vi "GetCollisions.vi"(8 "error in":errorcluster, 11 "sprite in":refnum<class "Sprite.lvclass">) -> (0 "error out":errorcluster, 2 "collisions out":string[](array[string]), 3 "sprite out":refnum<class "Sprite.lvclass">)   [LabVIEW 2010, in "RenderBase.lvlib" / "Sprite.lvclass"]
doc: "Returns the names of the objects that currently cause collisions. This is a default implementation that supports 2D collisions only. We also assume that the collisions don't change as long as the sprite's position doesn't change. Override this method if you need something more elaborated."
uses:
  Sprite.lvclass
  Sprite.lvclass/Sprite.ctl
  SceneObject_class/properties/SceneRoot/GetSceneRoot.vi
  SceneObject_class/properties/Position/GetPosition.vi
  SceneRoot_class/SceneRoot.lvclass
  SceneObject_class/SceneObject.lvclass
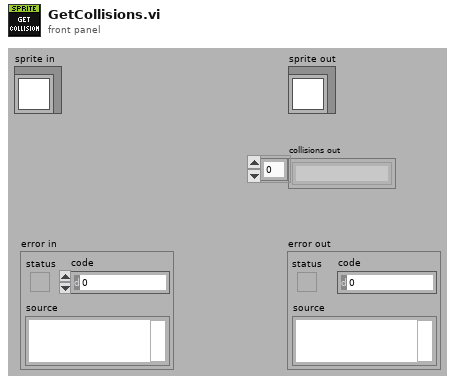
[diagram p1: front panel]
types:
  T1 = typedef "LV3DPointTypeDef.ctl" = cluster{"X":sgl, "Y":sgl, "Z":sgl}
  T2 = typedef "LVPoint32TypeDef.ctl" = cluster{"Horizontal":i32, "Vertical":i32}
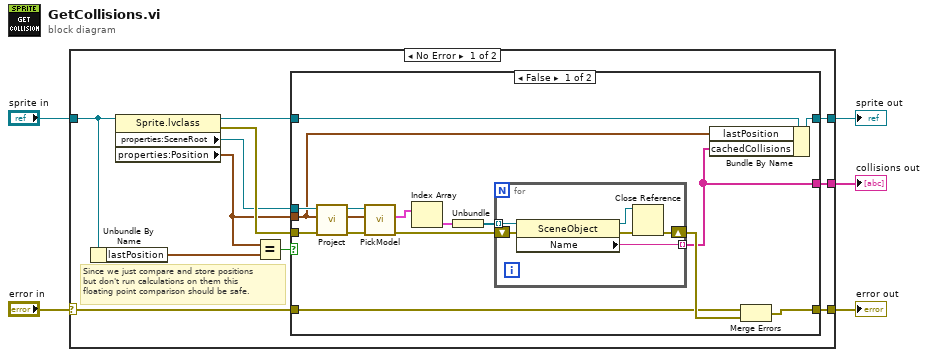
[diagram p0: block diagram]
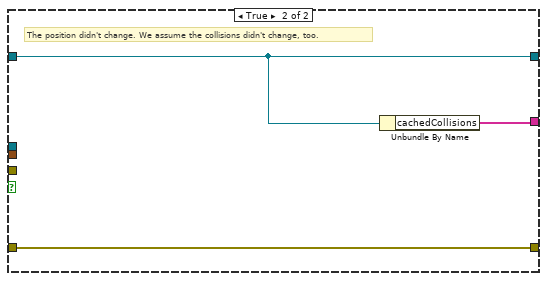
[diagram p2: hidden frame]
diagram:
  n1 = case shown="No Error" "error in" {
    selector: "error in" -> [w14 w43]
    tunnel: "sprite in" -> [w9 w42]
    tunnel: [w15 w43] -> w2
    tunnel: [w10 w42] -> w3
    tunnel: [w16 _] -> w4
    frame No Error {
      # "Since we just compare and store positions\nbut don't run calculations on them this\nfloating point comparison should be safe."
      n2 = Unbundle By Name(w9) -> ("lastPosition"=w6:T1)
      n3 = property class="Sprite.lvclass"(reference=w9) -> (reference out=w11:refnum<class "Sprite.lvclass">, error out=w13:errorcluster, "properties:SceneRoot"=w12:refnum<class "SceneRoot.lvclass">, "properties:Position"=w7:T1)  [unwired: 1 in]
      n4 = Equal?(x=w7, y=w6) -> (x = y?=w8:bool)
      n5 = case shown="False" w8 {
        tunnel: [w17 w40] -> w16
        tunnel: [w27 w39] -> w15
        tunnel: w14 -> [w26 w39]
        tunnel: w13 -> [w25 _]
        tunnel: w7 -> [w18 _]
        tunnel: w12 -> [w24 _]
        tunnel: w11 -> [w20 w41]
        tunnel: [w19 w41] -> w10
        frame False {
          n6 = call "Project.vi"("error in"=w25, "sceneCoords in"=w18, "class data in"=w24) -> ("error out"=w21:errorcluster, "winCoords out"=w22:T2, "class data out"=w23:refnum<class "SceneRoot.lvclass">)  [unwired: 6 in]
          n7 = call "PickModel.vi"("error in"=w21, "position in"=w22, "class data in"=w23) -> ("error out"=w28:errorcluster, "picked out"=w30:cluster{"Node Path":refnum<vi>[]}[])  [unwired: 6 in, 1 out]
          n8 = Index Array(array=w30) -> (element=w31:cluster{"Node Path":refnum<vi>[]})  [unwired: 1 in]
          n9 = Unbundle(w31) -> ("Node Path"=w32:refnum<vi>[])
          n10 = for {
            tunnel: w32 -> [w38] mode=indexing
            shift-right: [w33] -> w29
            shift-left: w28 -> [w37]
            tunnel: [w36] -> w17 mode=indexing
            n11 = property class="SceneObject"(reference=w38, error in=w37) -> (reference out=w34:refnum<vi>, error out=w35:errorcluster, "Name"=w36:string)
            n12 = Close Reference(reference=w34, error in (no error)=w35) -> (error out=w33:errorcluster)
          }
          n13 = Bundle By Name(cluster=w20, "lastPosition"=w18, "cachedCollisions"=w17) -> (w19:refnum<class "Sprite.lvclass">)
          n14 = Merge Errors(w26, w29) -> (w27:errorcluster)
        }
        frame True {
          # "The position didn't change. We assume the collisions didn't change, too."
          n15 = Unbundle By Name(w41) -> ("cachedCollisions"=w40:string[])
        }
      }
    }
    frame Error {
    }
  }
  "collisions out" <- w4
  "sprite out" <- w3
  "error out" <- w2
